vi "Read Msg Output.vi"(11 "Stopped Msg Output in":refnum<class "Stopped Msg Output.lvclass">) -> ()   [LabVIEW 2025, in "jettl.lvlib" / "Stopped jettl Msg.lvlib" / "Stopped Msg Output.lvlib" / "Stopped Msg Output.lvclass"]
uses:
  Stopped Msg Output.lvclass
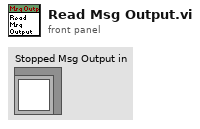
[diagram p1: front panel]
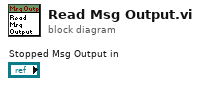
[diagram p0: block diagram]
diagram:
